vi "Sinconnect.vi"(0 "Start":dbl, 1 "dx/dy Start":dbl, 2 "Samples":dbl, 3 "End":dbl, 4 "dx/dy End":dbl) -> (5 "Sin Connection":dbl[](graph))   [LabVIEW 2015]
uses:
  <vilib>/Analysis/NI_AALBase.lvlib
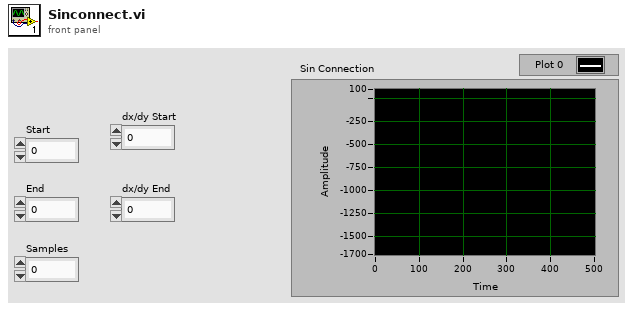
[diagram p1: front panel]
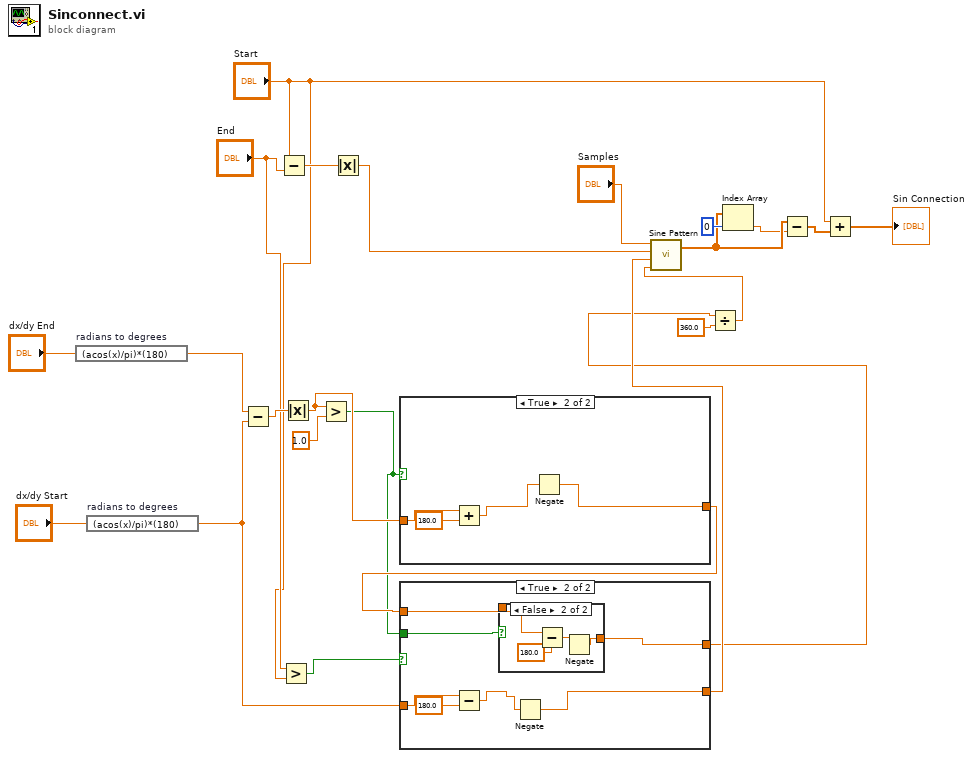
[diagram p0: block diagram]
diagram:
  n1 = expression code="(acos(x)/pi)*(180)" "radians to degrees"("dx/dy End") -> (w12:dbl)
  n2 = expression code="(acos(x)/pi)*(180)" "radians to degrees"("dx/dy Start") -> (w5:dbl)
  n3 = Subtract(x=w12, y=w5) -> (x-y=w10:dbl)
  n4 = Subtract(x="Start", y="End") -> (x-y=w21:dbl)
  n5 = Greater?(x="End", y="Start") -> (0:w6:bool)
  n6 = Absolute Value(x=w10) -> (abs(x)=w9:dbl)
  n7 = Greater?(x=w9, y=1.0) -> (0:w1:bool)
  n8 = Absolute Value(x=w21) -> (abs(x)=w20:dbl)
  n9 = case shown="True" w1 {
    tunnel: w9 -> [w25 w29]
    tunnel: [w25 w26] -> w3
    frame False {
    }
    frame True {
      n10 = Add(x=w29, y=180.0) -> (x+y=w27:dbl)
      n11 = Negate(x=w27) -> (-x=w26:dbl)
    }
  }
  n12 = case shown="True" w6 {
    tunnel: w5 -> [w31 w38]
    tunnel: [w31 w32] -> w4
    tunnel: w3 -> [w30 w36]
    tunnel: [w30 w35] -> w2
    tunnel: w1 -> [_ w34]
    frame False {
    }
    frame True {
      n13 = Subtract(x=w38, y=180.0) -> (x-y=w33:dbl)
      n14 = case shown="False" w34 {
        tunnel: w36 -> [w39 w43]
        tunnel: [w39 w40] -> w35
        frame True {
        }
        frame False {
          n15 = Subtract(x=w43, y=180.0) -> (x-y=w41:dbl)
          n16 = Negate(x=w41) -> (-x=w40:dbl)
        }
      }
      n17 = Negate(x=w33) -> (-x=w32:dbl)
    }
  }
  n18 = Divide(x=w2, y=360.0) -> (x/y=w23:dbl)
  n19 = call <vilib>:"Sine Pattern.vi"("cycles"=w23, "phase(degrees)"=w4, "amplitude"=w20, "samples"="Samples") -> ("Sinusoidal Pattern"=w18:dbl[])  [unwired: 1 out]
  n20 = Index Array(array=w18, index=0) -> (element=w17:dbl)
  n21 = Subtract(x=w18, y=w17) -> (x-y=w16:dbl[])
  n22 = Add(x="Start", y=w16) -> (x+y=→"Sin Connection":dbl[])
